vi "readSPEHeaderTest.vi"() -> ()   [LabVIEW 2015]
panel:
  in  "byte order":T1(ring)=enum."little-endian"
  in  "int offset":i64=4
  out "int":i16
  out "short":i8
  out "long":i32
  out "double":dbl
  out "error out":errorcluster caption="エラー出力"
  in  "error in":errorcluster caption="エラー入力"
  out "float":sgl
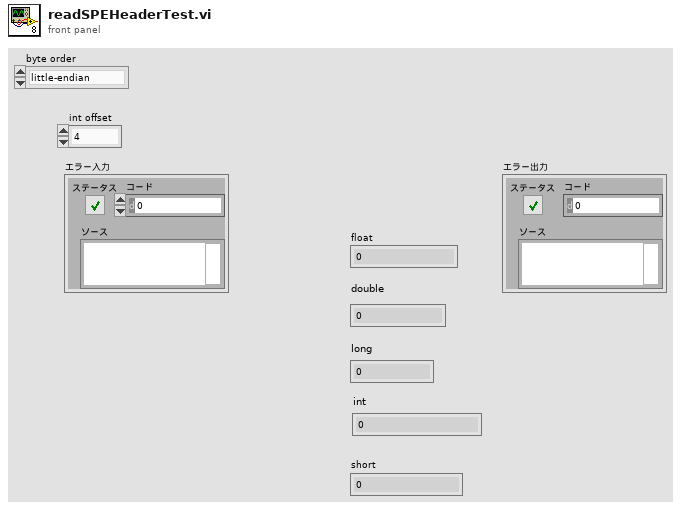
[diagram p1: front panel]
types:
  T1 = enum16{"big-endian, network order", "native, host order", "little-endian"}
  T2 = enum16{"open", "open or create", "create or replace", "create", "open (read only)"}
  T3 = enum16{"open", "replace", "create", "open or create", "replace or create", "replace or create with confirmation"}
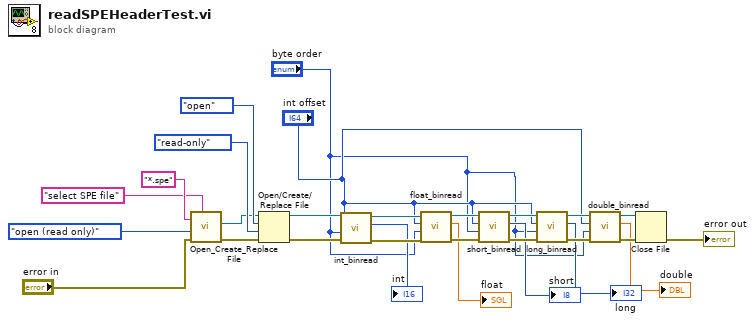
[diagram p0: block diagram]
diagram:
  n1 = call <vilib>:"Open_Create_Replace File.vi"("pattern"="*.spe", "prompt"="select SPE file", "error in (no error)"="error in", "function (open:0)"=T2."open (read only)") -> ("error out"=w24:errorcluster, "new file path"=w25:path)  [unwired: 4 in, 2 out]
  n2 = Open/Create/Replace File(file path (use dialog)=w25, error in=w24, operation (0:open)=T3."open", access (0:read/write)=enum16{"read/write", "read-only", "write-only"}."read-only" ("アクセス （0:read/write）")) -> (refnum out=w7:refnum<file>, error out=w4:errorcluster)  [unwired: 2 in, 1 out]
  n3 = call "int_binread.vi"("error in"=w4, "byte order"="byte order", "offset"="int offset", "ref in"=w7) -> ("error out"=w5:errorcluster, "int"=→"int":i16, "ref out"=w6:refnum<file>)  [unwired: 5 in]
  n4 = call "float_binread.vi"("error in"=w5, "byte order"="byte order", "offset"="int offset", "ref in"=w6) -> ("error out"=w13:errorcluster, "float"=→"float":sgl, "ref out"=w12:refnum<file>)  [unwired: 5 in]
  n5 = call "short_binread.vi"("error in"=w13, "byte order"="byte order", "offset"="int offset", "ref in"=w12) -> ("error out"=w20:errorcluster, "short"=→"short":i8, "ref out"=w21:refnum<file>)  [unwired: 5 in]
  n6 = call "long_binread.vi"("error in"=w20, "byte order"="byte order", "offset"="int offset", "ref in"=w21) -> ("error out"=w19:errorcluster, "long"=→"long":i32, "ref out"=w15:refnum<file>)  [unwired: 5 in]
  n7 = call "double_binread.vi"("error in"=w19, "byte order"="byte order", "offset"="int offset", "ref in"=w15) -> ("error out"=w18:errorcluster, "double"=→"double":dbl, "ref out"=w17:refnum<file>)  [unwired: 5 in]
  n8 = Close File(refnum=w17, error in=w18) -> (error out=→"error out":errorcluster)  [unwired: 1 out]
